vi "Keithley 6517 Read Temp and Humidity setup.vi"(6 "error in":T1, 9 "GPIB address":string="27") -> (0 "error out":T1)   [LabVIEW 2013]
doc: "This VI is used to read the primary and secondary display of the instrument. The primary display is selected from and of the function config VI's, while the secondary display is selected from the Disp2 Config VI."
panel:
  # "Run This VI ONCE after turning on Keithley  6517 Electro-sourcemeter\nto turn the 2nd front panel display to the temp & humidity reading"
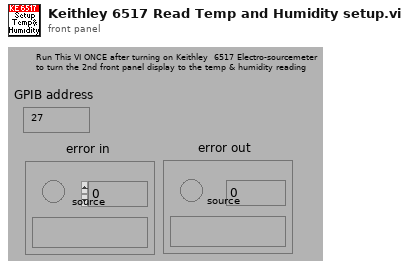
[diagram p1: front panel]
types:
  T1 = cluster{"error":bool, "code":i32, "source":string}
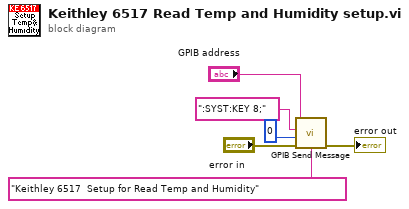
[diagram p0: block diagram]
diagram:
  n1 = call "GPIB Send Message.vi"("address string"="GPIB address", "write buffer"=":SYST:KEY 8;", "source"="Keithley 6517  Setup for Read Temp and Humidity", "write mode (set END:0)"=0, "error in"="error in") -> ("error out"=→"error out":T1)  [unwired: 2 in, 2 out]
